vi "I16_to_um_USB7855R.vi"(6 "-10 to 10V range?":bool, 8 "Max Value [um]":dbl, 9 "Channel Calibration":cluster{"LSB Weight":u32, "Offset":i32}, 11 "Input_I16":i16[](array[numeric])=[0, 0]) -> (2 "output_um":dbl[](array[numeric]))   [LabVIEW 2023]
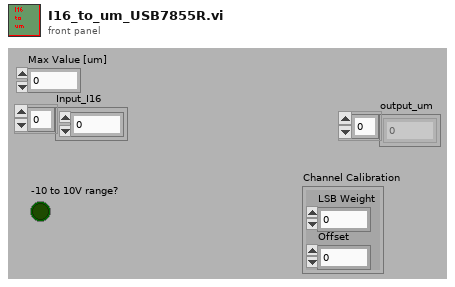
[diagram p1: front panel]
types:
  T1 = enum16{"USB 7855 (AI)", "USB 7855 (AO)", "USB 7855 OEM (AI)", "USB 7855 OEM (AO)", "USB 7856  (AI)", "USB 7856 (AO)", "USB 7856 OEM (AI)", "USB 7856 OEM (AO)"}
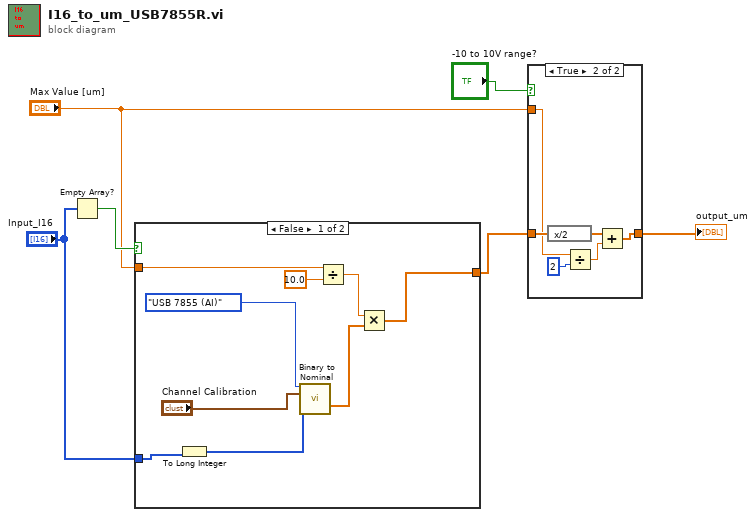
[diagram p0: block diagram]
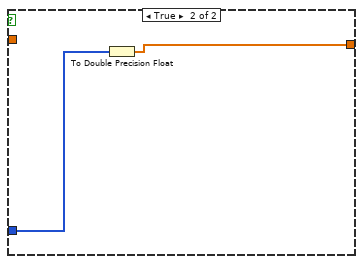
[diagram p3: hidden frame]
diagram:
  n1 = Empty Array?(array="Input_I16") -> (empty?=w5:bool)
  n2 = case shown="False" w5 {
    tunnel: "Input_I16" -> [w15 w17]
    tunnel: [w7 w16] -> w3
    tunnel: "Max Value [um]" -> [w11 _]
    frame False {
      n3 = To Long Integer(number=w15) -> (32bit integer=w14:i32[])
      n4 = call "Binary to Nominal.vi"("Target Type"=T1."USB 7855 (AI)", "Channel Calibration"="Channel Calibration", "Binary Value"=w14) -> ("Nominal Value"=w8:dbl[])  [unwired: 11 in, 1 out]
      n5 = Divide(x=w11, y=10.0) -> (x/y=w9:dbl)
      n6 = Multiply(x=w9, y=w8) -> (x*y=w7:dbl[])
    }
    frame True {
      n7 = To Double Precision Float(number=w17) -> (double precision float=w16:dbl[])
    }
  }
  n8 = case shown="True" "-10 to 10V range?" {
    tunnel: [w18 w20] -> w1
    tunnel: w3 -> [w18 w22]
    tunnel: "Max Value [um]" -> [_ w19]
    frame False {
    }
    frame True {
      n9 = expression code="x/2"(w22) -> (w21:dbl[])
      n10 = Divide(x=w19, y=2) -> (x/y=w23:dbl)
      n11 = Add(x=w21, y=w23) -> (x+y=w20:dbl[])
    }
  }
  "output_um" <- w1
